vi "Clousure.vi"(8 "error in (no error)":errorcluster, 11 "BombedWall":refnum<class "BombedWall.lvclass">) -> (0 "error out":errorcluster, 3 "BombedWall":refnum<class "BombedWall.lvclass">)   [LabVIEW 2020, in "BombedWall.lvclass"]
uses:
  BombedWall.lvclass
  Wall/Wall.lvclass
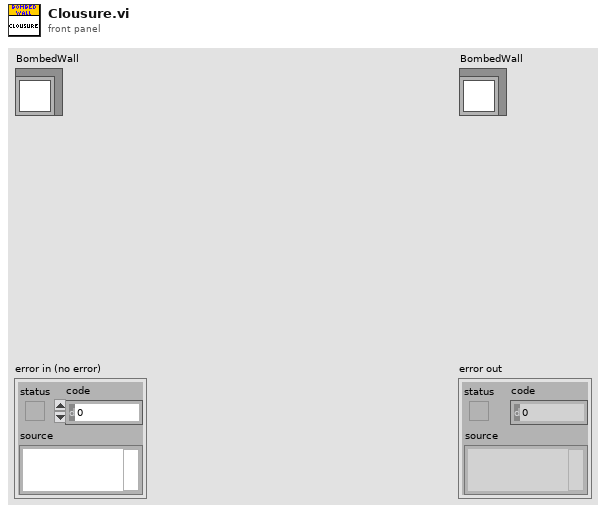
[diagram p1: front panel]
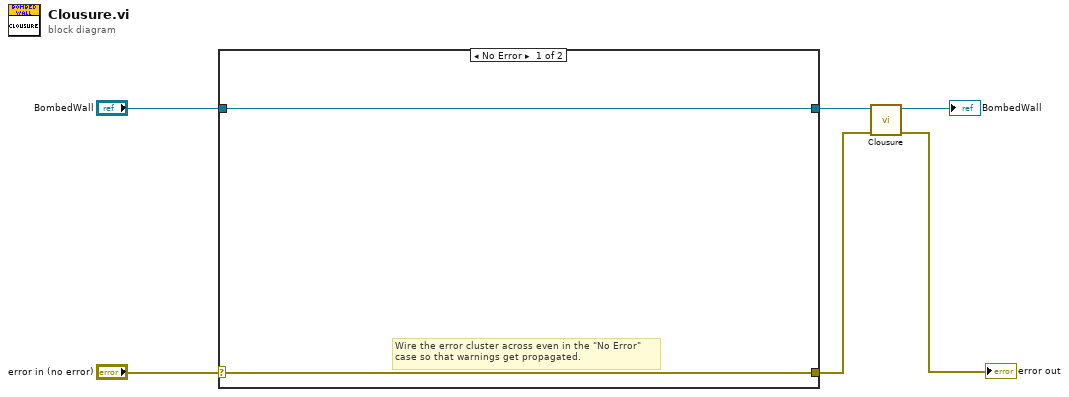
[diagram p0: block diagram]
diagram:
  n1 = case shown="No Error" "error in (no error)" {
    selector: "error in (no error)" -> [w7 w10]
    tunnel: [w7 w10] -> w2
    tunnel: [w8 w9] -> w4
    tunnel: "BombedWall" -> [w8 w9]
    frame No Error {
      # "Wire the error cluster across even in the \"No Error\"\ncase so that warnings get propagated."
    }
    frame Error {
    }
  }
  n2 = call-parent "Clousure.vi"("error in (no error)"=w2, "Wall"=w4) -> ("error out"=→"error out":errorcluster, "Wall"=→"BombedWall":refnum<class "BombedWall.lvclass">)  [unwired: 8 in]
